vi "Arm2Execute.vi"(8 "error in (no error)":errorcluster) -> (0 "error out":errorcluster)   [LabVIEW 2023]
doc: "Arm Execute for 2024 robot"
uses:
  <vilib>/Rock Robotics/WPI/ThirdParty/JAS_Junk/TrajLib/VI/BoolCmd_Recv_Internal.vi
  <vilib>/Rock Robotics/WPI/ThirdParty/JAS_Junk/TrajLib/VI/BoolCmd_ObtainQueue.vi
  <vilib>/Rock Robotics/Network Tables/NT Write Boolean.vi
  <vilib>/Rock Robotics/Network Tables/NT Write Number.vi
  Arm2Global.vi
  <vilib>/Rock Robotics/WPI/ThirdParty/JAS_Junk/TrajLib/Trajectory_Library.lvlib
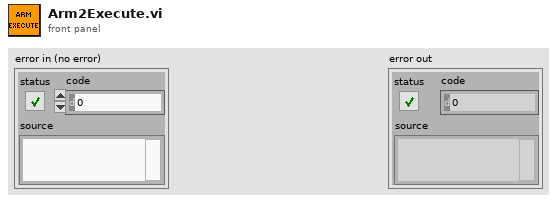
[diagram p1: front panel]
types:
  T1 = typedef "WPI_MotorControlDeviceRef.ctl" = cluster{"DeviceStatus":errorcluster, "Type":T2, "PWM":cluster{"PWM Channel":T3, "DeadBand":T4}, "CAN":cluster{"Device Number":u8, "SetOutput VI Ref":variant, "GetOutput VI Ref":variant, "Enable VI Ref":variant, "Disable VI Ref":variant, "Data":variant}, "Invert":bool, "DIO PWM":cluster{"PWM \"Enable\" Channel":T3, "DIOChannel":T5, "PWM Rate":dbl}}
  T2 = typedef "WPI_MotorControlType.ctl" = enum16{"PWM", "CAN", "DIO PWM"}
  T3 = typedef "FPGA_DIOPWMChannel.ctl" = enum8{"PWM 0", "PWM 1", "PWM 2", "PWM 3", "PWM 4", "PWM 5", "PWM 6", "PWM 7", "PWM 8", "PWM 9", "PWM MXP 0", "PWM MXP 1", "PWM MXP 2", "PWM MXP 3", "PWM MXP 4", "PWM MXP 5", "PWM MXP 6", "PWM MXP 7", "PWM MXP 8", "PWM MXP 9", "Invalid"}
  T4 = typedef "WPI_PWMDeadband.ctl" = cluster{"Name":string, "maxPositivePwm":i32, "minPositivePwm":i32, "centerPwm":i32, "maxNegativePwm":i32, "minNegativePwm":i32, "angularRange":u16}
  T5 = typedef "FPGA_DIOChannel.ctl" = enum8{"DIO 0", "DIO 1", "DIO 2", "DIO 3", "DIO 4", "DIO 5", "DIO 6", "DIO 7", "DIO 8", "DIO 9", "DIO MXP 0", "DIO MXP 1", "DIO MXP 2", "DIO MXP 3", "DIO MXP 4", "DIO MXP 5", "DIO MXP 6", "DIO MXP 7", "DIO MXP 8", "DIO MXP 9", "DIO MXP 10", "DIO MXP 11", "DIO MXP 12", "DIO MXP 13", "DIO MXP 14", "DIO MXP 15", "SPI Port CS1", "SPI Port CS2", "SPI Port CS3", "SPI Port MISO", "SPI Port MOSI", "Invalid"}
  T6 = typedef "Trajectory_Library.lvlib/PosCtrl_Tuning_Type.ctl" = cluster{"Slope":dbl, "Offset":dbl, "Error Deadband":dbl, "At Reference Count":i32, "Negate Output":bool, "Max Allowd Position":dbl, "Min Allowd Position":dbl}
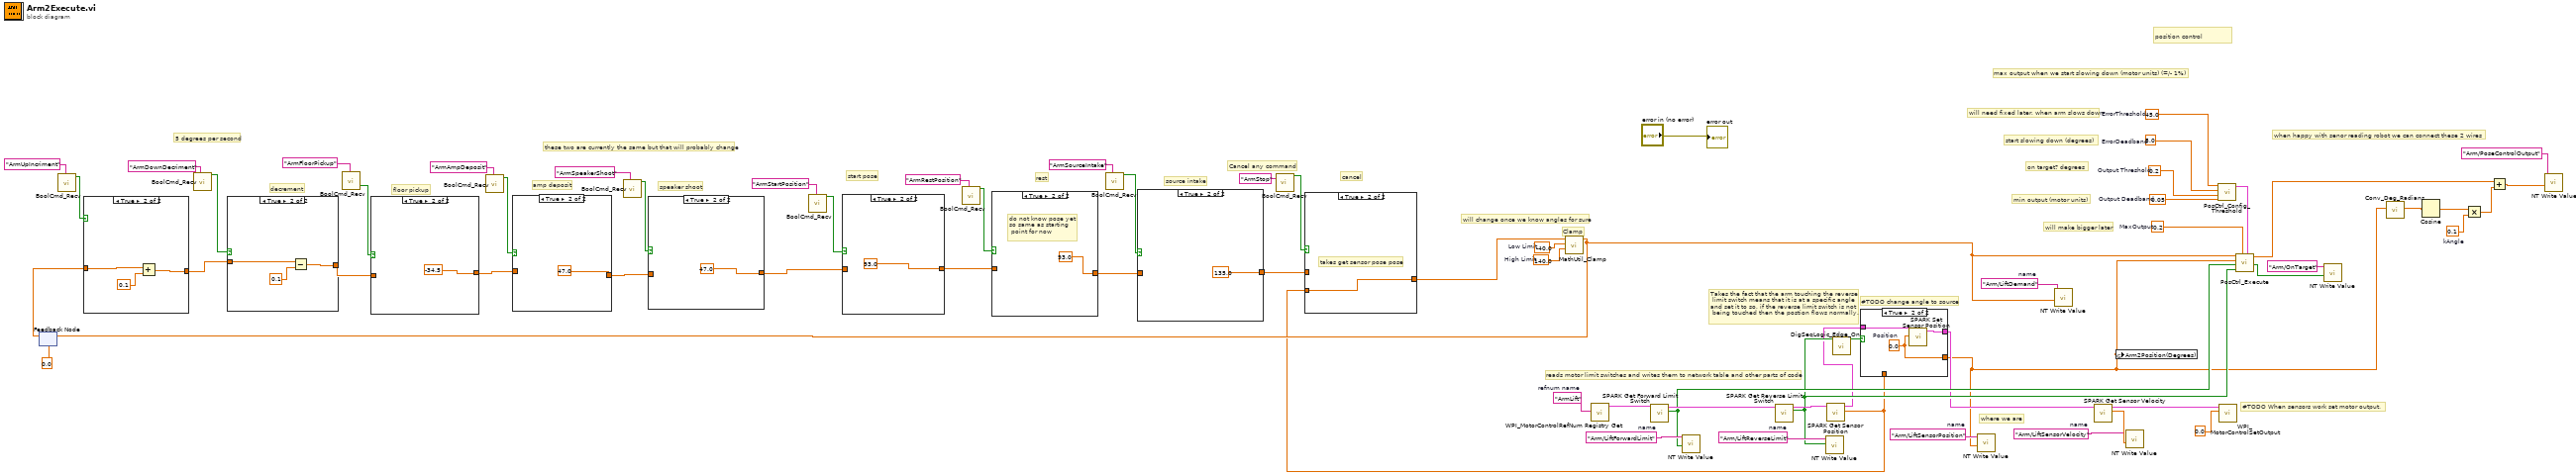
[diagram p0: block diagram]
diagram:
  w5 = 0.1  # kAngle
  w37 = 140.0  # High Limit
  w36 = -40.0  # Low Limit
  w51 = "Arm/LiftDemand"  # name
  w53 = "Arm/LiftSensorVelocity"  # name
  w54 = "Arm/LiftSensorPosition"  # name
  w55 = "Arm/LiftReverseLimit"  # name
  w56 = "Arm/LiftForwardLimit"  # name
  w58 = "ArmLift"  # refnum name
  w67 = 0.2  # MaxOutput
  w65 = 45.0  # ErrorThreshold
  w64 = 5.0  # ErrorDeadband
  w63 = 0.2  # Output Threshold
  w62 = 0.05  # Output Deadband
  # "these two are currently the same but that will probably change"
  # "Cancel any command"
  # "source intake"
  # "will change once we know angles for sure"
  # "cancel"
  # "rest"
  # "start pose"
  # "speaker shoot"
  # "Clamp"
  # "5 degrees per second"
  # "amp deposit"
  # "floor pickup"
  # "decrement"
  # "#TODO change angle to source"
  # "Takes the fact that the arm touching the reverse\n limit switch means that it is at a specific angle \nand set it to so, if the reverse limit switch is not\n being touched then the postion flows normally."
  # "#TODO When sensors work set motor output."
  # "when happy with senor reading robot we can connect these 2 wires"
  # "min output (motor units)"
  # "max output when we start slowing down (motor units) (=/- 1%)"
  # "on target? degrees"
  # "start slowing down (degrees)"
  # "will make bigger later"
  # "where we are"
  # "position control"
  # "will need fixed later, when arm slows down"
  # "reads motor limit switches and writes them to network table and other parts of code"
  n1 = feedback #1(0.0 ("Result")) -> (w41:dbl)
  n2 = call <vilib>:"BoolCmd_Recv.vi"("Command Name"="ArmUpIncriment") -> ("New Request"=w28:bool)  [unwired: 9 in, 1 out]
  n3 = case shown="True" w28 {
    tunnel: w41 -> [w68 w71]
    tunnel: [w68 w69] -> w40
    frame False {
    }
    frame True {
      n4 = Add(x=w71, y=0.1) -> (x+y=w69:dbl)
    }
  }
  n5 = call <vilib>:"BoolCmd_Recv.vi"("Command Name"="ArmDownDecriment") -> ("New Request"=w26:bool)  [unwired: 9 in, 1 out]
  n6 = case shown="True" w26 {
    tunnel: w40 -> [w72 w74]
    tunnel: [w72 w73] -> w39
    frame False {
    }
    frame True {
      n7 = Subtract(x=w74, y=0.1) -> (x-y=w73:dbl)
    }
  }
  n8 = call <vilib>:"BoolCmd_Recv.vi"("Command Name"="ArmFloorPickup") -> ("New Request"=w24:bool)  [unwired: 9 in, 1 out]
  n9 = case shown="True" w24 {
    tunnel: w39 -> [w76 _]
    tunnel: [w76 -34.5 ("y")] -> w38
    frame False {
    }
    frame True {
    }
  }
  n10 = call <vilib>:"BoolCmd_Recv.vi"("Command Name"="ArmAmpDeposit") -> ("New Request"=w22:bool)  [unwired: 9 in, 1 out]
  n11 = case shown="True" w22 {
    tunnel: w38 -> [w78 _]
    tunnel: [w78 47.0 ("y")] -> w35
    frame False {
    }
    frame True {
    }
  }
  n12 = call <vilib>:"BoolCmd_Recv.vi"("Command Name"="ArmSpeakerShoot") -> ("New Request"=w20:bool)  [unwired: 9 in, 1 out]
  n13 = case shown="True" w20 {
    tunnel: w35 -> [w80 _]
    tunnel: [w80 47.0 ("y")] -> w34
    frame False {
    }
    frame True {
    }
  }
  n14 = call <vilib>:"BoolCmd_Recv.vi"("Command Name"="ArmStartPosition") -> ("New Request"=w18:bool)  [unwired: 9 in, 1 out]
  n15 = case shown="True" w18 {
    tunnel: w34 -> [w82 _]
    tunnel: [w82 93.0 ("y")] -> w33
    frame False {
    }
    frame True {
    }
  }
  n16 = call <vilib>:"BoolCmd_Recv.vi"("Command Name"="ArmRestPosition") -> ("New Request"=w16:bool)  [unwired: 9 in, 1 out]
  n17 = case shown="True" w16 {
    tunnel: w33 -> [w84 _]
    tunnel: [w84 93.0 ("y")] -> w32
    frame False {
    }
    frame True {
      # "do not know pose yet \nso same as starting\n point for now"
    }
  }
  n18 = call <vilib>:"BoolCmd_Recv.vi"("Command Name"="ArmSourceIntake") -> ("New Request"=w14:bool)  [unwired: 9 in, 1 out]
  n19 = case shown="True" w14 {
    tunnel: w32 -> [w86 _]
    tunnel: [w86 135.0 ("y")] -> w31
    frame False {
    }
    frame True {
    }
  }
  n20 = call <vilib>:"BoolCmd_Recv.vi"("Command Name"="ArmStop") -> ("New Request"=w12:bool)  [unwired: 9 in, 1 out]
  n21 = call <vilib>:"WPI_MotorControlRefNum Registry Get.vi"("refnum name"=w58) -> ("MotorControlDevRef"=w61:T1)  [unwired: 9 in, 1 out]
  n22 = call <vilib>:"SPARK Get Forward Limit Switch.vi"("MotorControlDevRef in"=w61) -> ("Hard Limit Fwd"=w52:bool, "MotorControlDevRef out"=w59:T1)  [unwired: 7 in, 2 out]
  n23 = call-poly <vilib>:"NT Write Value.vi"("value"=w52, "name"=w56) -> ()  [unwired: 9 in, 1 out]
  n24 = call <vilib>:"SPARK Get Reverse Limit Switch.vi"("MotorControlDevRef in"=w59) -> ("Hard Limit Rev"=w45:bool, "MotorControlDevRef out"=w60:T1)  [unwired: 7 in, 2 out]
  n25 = call-poly <vilib>:"NT Write Value.vi"("value"=w45, "name"=w55) -> ()  [unwired: 9 in, 1 out]
  n26 = call <vilib>:"SPARK Get Sensor Position.vi"("MotorControlDevRef in"=w60) -> ("Sensor Position"=w9:dbl, "MotorControlDevRef out"=w43:T1)  [unwired: 7 in, 2 out]
  n27 = case shown="True" w12 {
    tunnel: w31 -> [w88 _]
    tunnel: [w88 w89] -> w30
    tunnel: w9 -> [_ w89]
    frame False {
    }
    frame True {
      # "takes get sensor pose pose"
    }
  }
  n28 = call <vilib>:"MathUtil_Clamp.vi"("High Limit"=w37, "Low Limit"=w36, "Value"=w30) -> ("Result"=w11:dbl)  [unwired: 8 in]
  n29 = feedback-in #1(w11) -> ()
  n30 = call <vilib>:"DigSeqLogic_Edge_On.vi"("Input"=w45) -> ("On Edge"=w44:bool)  [unwired: 10 in]
  n31 = case shown="True" w44 {
    tunnel: w43 -> [w90 w94]
    tunnel: [w90 w93] -> w42
    tunnel: [w91 w92] -> w1
    tunnel: w9 -> [w91 _]
    frame False {
    }
    frame True {
      w92 = 0.0  # Position
      n32 = call <vilib>:"SPARK Set Sensor Position.vi"("Position"=w92, "MotorControlDeviceRef"=w94) -> ("MotorControlDeviceRef"=w93:T1)  [unwired: 8 in, 1 out]
    }
  }
  n33 = call-poly <vilib>:"NT Write Value.vi"("value"=w1, "name"=w54) -> ()  [unwired: 9 in, 1 out]
  n34 = call-poly <vilib>:"NT Write Value.vi"("value"=w11, "name"=w51) -> ()  [unwired: 9 in, 1 out]
  n35 = call <vilib>:"SPARK Get Sensor Velocity.vi"("MotorControlDevRef in"=w42) -> ("Sensor Velocity"=w57:dbl, "MotorControlDevRef out"=w49:T1)  [unwired: 7 in, 2 out]
  n36 = global write "Arm2Global.vi" "Arm2Position(Degrees)"(w1) -> ()
  n37 = call-poly <vilib>:"NT Write Value.vi"("value"=w57, "name"=w53) -> ()  [unwired: 9 in, 1 out]
  n38 = call <vilib>:"PosCtrl_Config_Threshold.vi"("Output Deadband"=w62, "Output Threshold"=w63, "ErrorDeadband"=w64, "ErrorThreshold"=w65) -> ("PosCtrl_Config_Params"=w66:T6)  [unwired: 7 in]
  n39 = call <vilib>:"WPI_MotorControlSetOutput.vi"("Output"=0.0, "MotorControlDevRef"=w49) -> ()  [unwired: 7 in, 3 out]
  n40 = call <vilib>:"PosCtrl_Execute.vi"("PosCtrl_Config_Params"=w66, "MaxOutput"=w67, "Rev Limit Switch"=w45, "Fwd Limit Switch"=w52, "CurrentPosition"=w1, "TargetPosition"=w11) -> ("OnTarget"=w48:bool, "Output"=w7:dbl)  [unwired: 3 in, 1 out]
  n41 = call-poly <vilib>:"NT Write Value.vi"("value"=w48, "name"="Arm/OnTarget") -> ()  [unwired: 9 in, 1 out]
  n42 = call <vilib>:"Conv_Deg_Radians.vi"("Degress"=w1) -> ("Radians"=w2:dbl)  [unwired: 10 in]
  n43 = Cosine(x=w2) -> (cos(x)=w4:dbl)
  n44 = Multiply(x=w4, y=w5) -> (x*y=w6:dbl)
  n45 = Add(x=w7, y=w6) -> (x+y=w3:dbl)
  n46 = call-poly <vilib>:"NT Write Value.vi"("value"=w3, "name"="Arm/PoseControlOutput") -> ()  [unwired: 9 in, 1 out]
  "error out" <- "error in (no error)"
